vi "ExperimentStateStore.vi"(2 "error in":errorcluster, 3 "Experiment State":T1={"error"={"status"=FALSE, "code"=0, "source"=""}, "Digitizer DAQmx Tasks"={"TaskArray"=[]}, "Digitizer Settings"={"Channel Settings"=[], "Card Settings"=[]}, "Synchronization Settings"={"Synchronizer"="PXI1Slot2", "source terminal"="GlobalSoftwareTrigger"}, "Digitizer Data"=[], "Next Shot#"="0", "System Message"="", "User Shot Notes"="", "Timing Settings"={"Timing Card Settings"=[], "Timing Channel Settings"=[[{"Delay (s)"=2.559999942779541, "Pulse width (s)"=0.009999999776482582, "Active"=TRUE, "Channel Name"="Fiber 8", "counter"="PXI1Slot8/ctr7"}]]}, "Timing Tasks"={"TaskArray"=[]}} {"Timing Settings"."Timing Channel Settings"."Pulse width (s)" format="%.3p"; "Timing Settings"."Timing Channel Settings"."Delay (s)" format="%.3p"; "Digitizer Settings"."Card Settings"."Global Edge Type" items=["Rising"=10280, "Falling"=10171]; "Digitizer Settings"."Card Settings"."Sample Rate" format="%#_3p"}, 4 "Tree name":string="proto_tree") -> (0 "Error Message":errorcluster)   [LabVIEW 2013]
uses:
  Controls/ExperimentStateCluster.ctl
  Controls/DigitizerSettingsChannelSettings.ctl
  Controls/DigitizerSettingsCardSettingsArray.ctl
  Controls/DigitizerSettingsCardSettings.ctl
  Controls/TimingCardSettings.ctl
  Controls/TimingChannelSettings.ctl
  <vilib>/MDSplus/Library/MDSplus.lvlib
  <vilib>/MDSplus/Classes/Tree_Class/Tree.lvclass
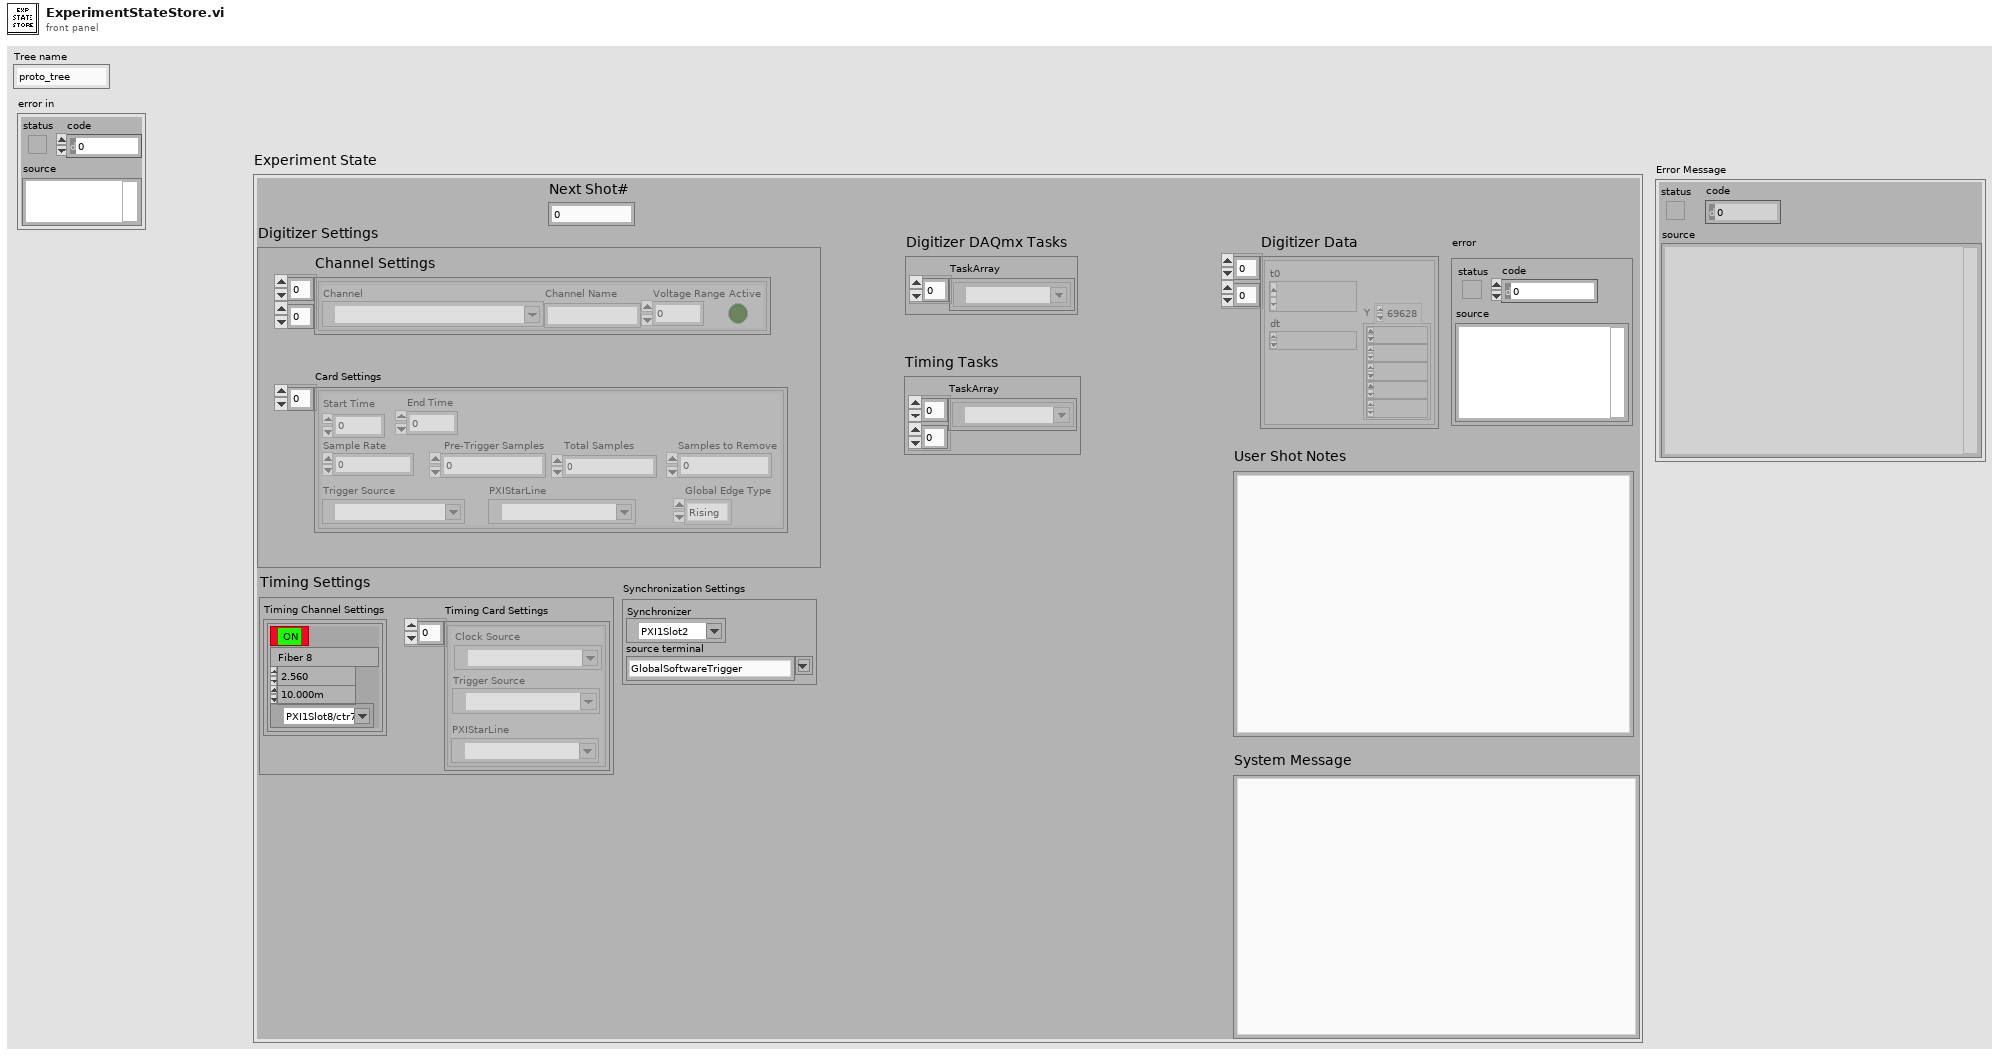
[diagram p1: front panel]
types:
  T1 = typedef "ExperimentStateCluster.ctl" = cluster{"error":errorcluster, "Digitizer DAQmx Tasks":cluster{"TaskArray":refnum<k21>[]}, "Digitizer Settings":cluster{"Channel Settings":T2[][], "Card Settings":T3}, "Synchronization Settings":cluster{"Synchronizer":refnum<k15>, "source terminal":string}, "Digitizer Data":waveform(dbl)[][], "Next Shot#":string, "System Message":string, "User Shot Notes":string, "Timing Settings":cluster{"Timing Card Settings":T5[], "Timing Channel Settings":T6[][]}, "Timing Tasks":cluster{"TaskArray":refnum<k21>[][]}}
  T2 = typedef "DigitizerSettingsChannelSettings.ctl" = cluster{"Channel":tag, "Channel Name":string, "Voltage Range":dbl, "Active":bool}
  T3 = typedef "DigitizerSettingsCardSettingsArray.ctl" = T4[]
  T4 = typedef "DigitizerSettingsCardSettings.ctl" = cluster{"Start Time":dbl, "End Time":dbl, "Sample Rate":dbl, " Pre-Trigger Samples":u32, "Total Samples":i32, "Samples to Remove":u32, "Trigger Source":tag, "Global Edge Type":i32, "PXIStarLine":tag}
  T5 = typedef "TimingCardSettings.ctl" = cluster{"Trigger Source":tag, "Clock Source":tag, "PXIStarLine":tag}
  T6 = typedef "TimingChannelSettings.ctl" = cluster{"Delay (s)":dbl, "Pulse width (s)":dbl, "Active":bool, "Channel Name":string, "counter":tag}
  T7 = cluster{"Channel Settings":T2[][], "Card Settings":T3}
  T8 = cluster{"Timing Card Settings":T5[], "Timing Channel Settings":T6[][]}
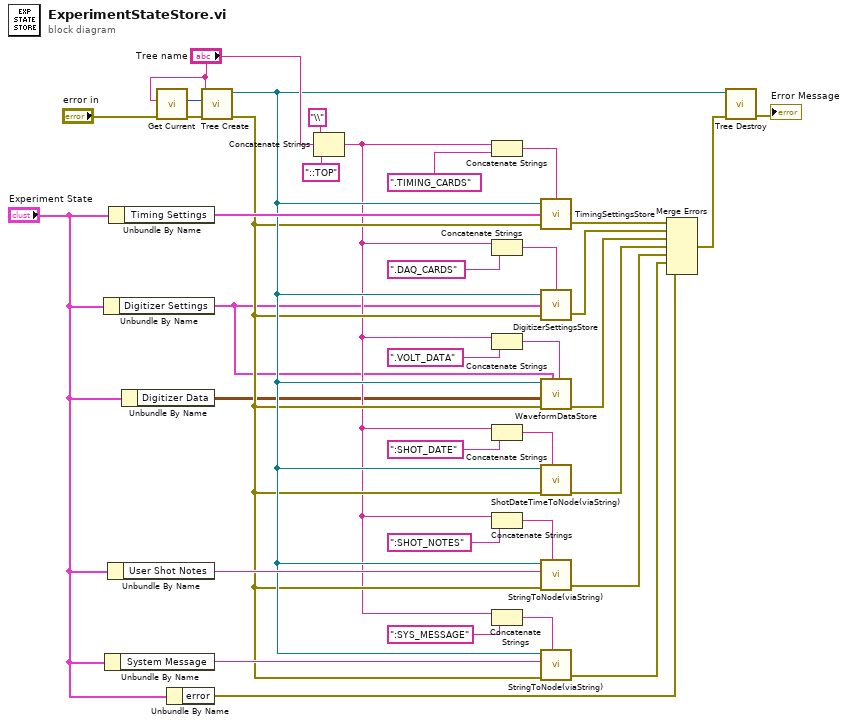
[diagram p0: block diagram]
diagram:
  n1 = Unbundle By Name("Experiment State") -> ("Digitizer Settings"=w3:T7)
  n2 = Unbundle By Name("Experiment State") -> ("System Message"=w16:string)
  n3 = Unbundle By Name("Experiment State") -> ("User Shot Notes"=w19:string)
  n4 = Unbundle By Name("Experiment State") -> ("Timing Settings"=w20:T8)
  n5 = Unbundle By Name("Experiment State") -> ("Digitizer Data"=w4:waveform(dbl)[][])
  n6 = call <vilib>:"Get Current.vi"("error in (no error)"="error in", "Tree name"="Tree name") -> ("error out"=w35:errorcluster, "Current shot out"=w36:i32)  [unwired: 7 in, 1 out]
  n7 = Unbundle By Name("Experiment State") -> ("error"=w12:errorcluster)
  n8 = call <vilib>:"Tree Create.vi"("error in (no error)"=w35, "Shot"=w36, "Name"="Tree name") -> ("error out"=w9:errorcluster, "Tree DVR out"=w10:refnum<data-value>)  [unwired: 7 in]
  n9 = Concatenate Strings("\\" ("string"), "Tree name", "::TOP" ("string")) -> (w5:string)
  n10 = Concatenate Strings(w5, ".TIMING_CARDS" ("string")) -> (w21:string)
  n11 = Concatenate Strings(w5, ".DAQ_CARDS" ("string")) -> (w23:string)
  n12 = Concatenate Strings(w5, ".VOLT_DATA") -> (w11:string)
  n13 = Concatenate Strings(w5, ":SHOT_DATE") -> (w27:string)
  n14 = Concatenate Strings(w5, ":SHOT_NOTES" ("NodePath")) -> (w25:string)
  n15 = Concatenate Strings(w5, ":SYS_MESSAGE" ("NodePath")) -> (w17:string)
  n16 = call "TimingSettingsStore.vi"("Tree Path In"=w21, "error in"=w9, "Timing Settings"=w20, "Tree DVR In"=w10) -> ("error out"=w7:errorcluster)  [unwired: 1 in]
  n17 = call "DigitizerSettingsStore.vi"("Tree Path In"=w23, "error in"=w9, "Digitizer Settings"=w3, "Tree DVR In"=w10) -> ("error out"=w6:errorcluster)  [unwired: 1 in]
  n18 = call "WaveformDataStore.vi"("Digitizer Settings"=w3, "error in"=w9, "Digitizer Data"=w4, "Tree Path In"=w11, "Tree DVR In"=w10) -> ("error out"=w8:errorcluster)  [unwired: 6 in]
  n19 = call "ShotDateTimeToNode(viaString).vi"("DateTime Path"=w27, "error in"=w9, "Tree DVR in"=w10) -> ("error out"=w15:errorcluster)  [unwired: 8 in]
  n20 = call "StringToNode(viaString).vi"("Tree DVR in"=w10, "String value in"=w19, "error in (no error)"=w9, "NodePath"=w25) -> ("error out"=w14:errorcluster)  [unwired: 1 in, 2 out]
  n21 = call "StringToNode(viaString).vi"("Tree DVR in"=w10, "String value in"=w16, "error in (no error)"=w9, "NodePath"=w17) -> ("error out"=w13:errorcluster)  [unwired: 1 in, 2 out]
  n22 = Merge Errors(w7, w6, w8, w15, w14, w13, w12) -> (w33:errorcluster)
  n23 = call <vilib>:"Tree Destroy.vi"("error in (no error)"=w33, "Tree DVR in"=w10) -> ("error out"=→"Error Message":errorcluster)  [unwired: 9 in]
